vi "Write Text.vi"(8 "error in (no error)":errorcluster, 9 "timeout ms (5000)":i32=5000, 10 "String Data":string, 11 "WebSocket in":refnum<class "WebSocket.lvclass">) -> (0 "error out":errorcluster, 3 "WebSocket out":refnum<class "WebSocket.lvclass">)   [LabVIEW 2021, in "WebSockets.lvlib" / "WebSocket.lvclass"]
doc: "Writes a text frame to the WebSocket connection endpoint.\nWebSockets 2.0.1.40\nSam Sharp - MediaMongrels Ltd\nCopyright (c) 2019, MediaMongrels Ltd"
uses:
  WebSocket.lvclass
  Opcodes.ctl
  WebSocket.lvclass/WebSocket.ctl
  DataLengthBytes.vi
  EncodeMaskedBytes.vi
  Socket Write.vi
  Sockets/Socket/Socket.lvclass
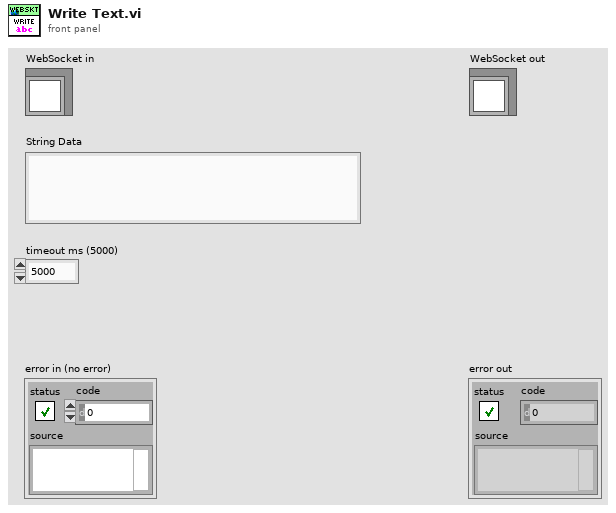
[diagram p1: front panel]
types:
  T1 = typedef "WebSockets.lvlib/WebSocket.lvclass/Opcodes.ctl" = u8
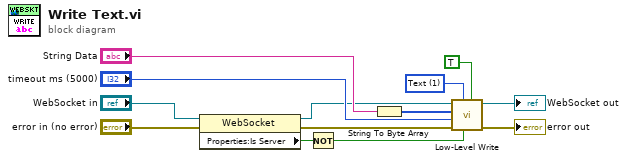
[diagram p0: block diagram]
diagram:
  w1 = T1 1 items=["Cont. Frame"=0, "Text"=1, "Binary"=2, "Close Frame"=8, "Ping"=9, "Pong"=10] ("Opcode (Text)")
  n1 = property class="WebSocket"(reference="WebSocket in", error in="error in (no error)") -> (reference out=w6:refnum<class "WebSocket.lvclass">, error out=w4:errorcluster, "Properties:Is Server"=w3:bool)
  n2 = Not(x=w3) -> (.not. x?=w2:bool)
  n3 = String To Byte Array(string="String Data") -> (unsigned byte array=w8:u8[])
  n4 = call "Low-Level Write.vi"("Finished? (True)"=TRUE, "Mask payload?"=w2, "Opcode (Text)"=w1, "error in (no error)"=w4, "timeout ms (5000)"="timeout ms (5000)", "Data"=w8, "WebSockets in"=w6) -> ("error out"=→"error out":errorcluster, "WebSockets out"=→"WebSocket out":refnum<class "WebSocket.lvclass">)  [unwired: 2 in, 1 out]
